vi "Serial_Enumerate Ports.vi"(11 "Python version":string="3.9") -> (0 "error out":errorcluster, 1 "guess":string, 3 "Python":T1, 5 "possibilities":string[](array[string]))   [LabVIEW 2020]
uses:
  PythonCtrl.ctl
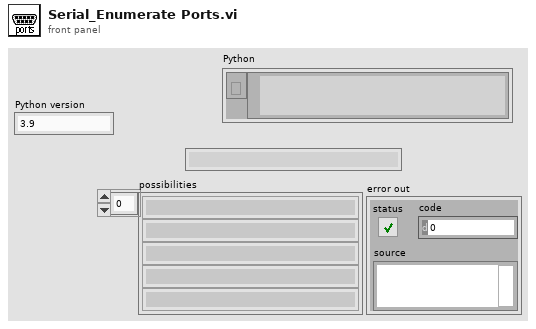
[diagram p1: front panel]
types:
  T1 = typedef "PythonCtrl.ctl" = cluster{"session":refnum<k35>, "PyPath":path}
  T2 = cluster{"session out":refnum<k35>, "appended path":path}
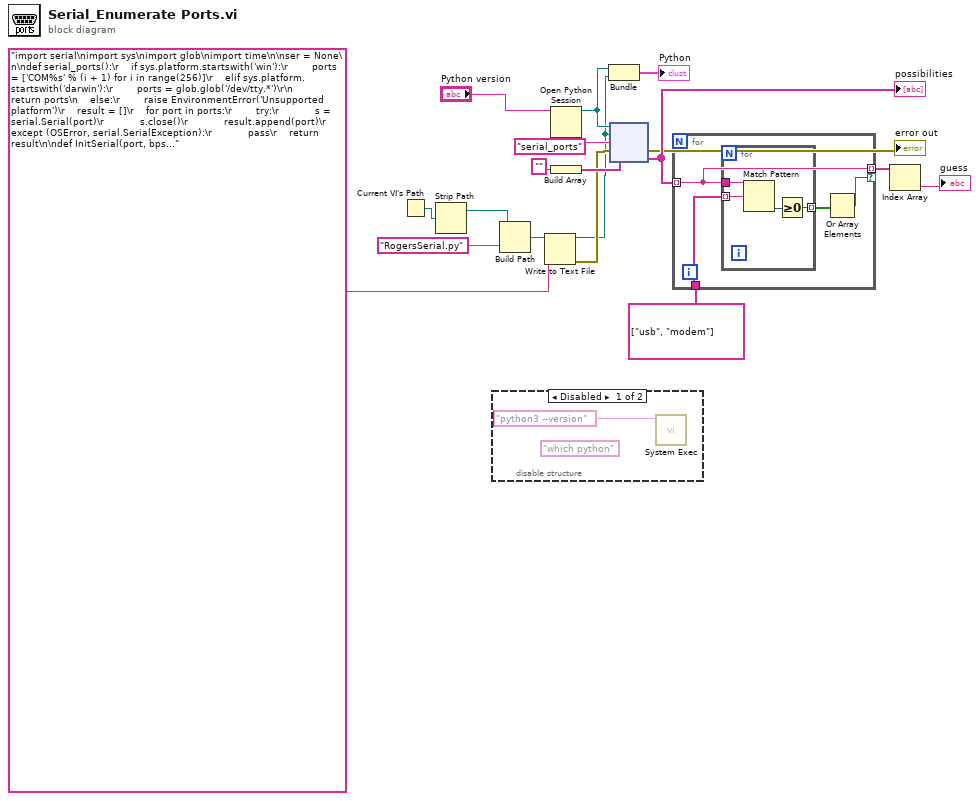
[diagram p0: block diagram]
diagram:
  n1 = Current VI's Path() -> (path=w9:path)
  n2 = Strip Path(path=w9) -> (stripped path=w8:path)  [unwired: 1 out]
  n3 = disable-structure shown="Disabled" {
    frame Disabled {
      (unwired) "which python" ("command line")
      n4 = call <vilib>:"System Exec.vi"("command line"="python3 --version") -> ()  [unwired: 7 in, 4 out]
    }
    frame Enabled {
    }
  }
  n5 = Build Path(base path=w8, name or relative path="RogersSerial.py") -> (appended path=w2:path)
  n6 = Write to Text File(file (use dialog)=w2, text="import serial\nimport sys\nimport glob\nimport time\n\nser = None\n\ndef serial_ports():\r    if sys.platform.startswith('win'):\r        ports = ['COM%s' % (i + 1) for i in range(256)]\r    elif sys.platform.startswith('darwin'):\r        ports = glob.glob('/dev/tty.*')\r\n        return ports\n    else:\r        raise EnvironmentError('Unsupported platform')\r    result = []\r    for port in ports:\r        try:\r            s = serial.Serial(port)\r            s.close()\r            result.append(port)\r        except (OSError, serial.SerialException):\r            pass\r    return result\n\ndef InitSerial(port, bps = 9600, to = 0):\n    global ser\n    ser = serial.Serial(port, bps, timeout = to)  # open serial port\n    return (ser.name)\n\ndef CloseSerial():\n    global ser\n    ser.close()\n    return('done')\n\ndef WriteSerial(string):\n    global ser\n    return(ser.write(string.encode()))    # write a string\n\ndef ScriptSerial(string):\n    global ser\n    reply = ''\n    lines = string.split('\\n')\n    for line in lines:\n        ser.write(line.encode())\n        time.sleep(1)\n        reply += ReadSerial() + '\\n'\n    return reply \n\ndef ReadSerial():\n    global ser\n    reply = ''\n    if ser.in_waiting:\n        reply = ser.readline().decode()\n    return(reply)\n") -> (error out=w7:errorcluster)  [unwired: 2 in, 2 out]
  n7 = Open Python Session(python version="Python version") -> (session out=w3:refnum<k35>)  [unwired: 2 in, 1 out]
  n8 = Build Array("" ("function name")) -> (w12:string[])
  n9 = Bundle("session out"=w3, "appended path"=w2) -> (→"Python":T2)  [unwired: 1 in]
  n10 = node(w3, w2, "serial_ports" ("function name"), w7, w12) -> (→"error out":errorcluster, w5:string[])  [unwired: 3 out]
  "possibilities" <- w5
  n11 = for {
    tunnel: w5 -> [w20] mode=indexing
    tunnel: string[] ["usb", "modem"] -> [w22]
    tunnel: [w20] -> w16 mode=indexing if=w19
    n12 = for {
      tunnel: w20 -> [w26]
      tunnel: w22 -> [w25] mode=indexing
      tunnel: [w23] -> w21 mode=indexing
      n13 = Match Pattern(string=w26, regular expression=w25) -> (offset past match=w24:i32)  [unwired: 1 in, 3 out]
      n14 = Greater Or Equal To 0?(x=w24) -> (x >= 0?=w23:bool)
    }
    n15 = Or Array Elements(Boolean array=w21) -> (logical OR=w19:bool)
  }
  n16 = Index Array(array=w16) -> (element=→"guess":string)  [unwired: 1 in]
